vi "commCAS.vi"() -> ()   [LabVIEW 2021]
panel:
  in  "CommCAS":dbl
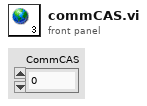
[diagram p1: front panel]
diagram:
